vi "ReadINI.vi"(8 "error in (no error)":errorcluster) -> (0 "error out":errorcluster, 3 "value":T1={"TrackQueues?"=TRUE, "ClientTimeout (s)"=30, "LogPath"=path "", "ErrorsToIgnore"=[], "OracleData"={"DBname"="", "User"="", "Password"=""}})   [LabVIEW 2017, in "Server.lvlib"]
uses:
  Server.lvlib
  TypeDefs/ServerINI.ctl
  SubLibs/Oracle/OracleData.ctl
  <vilib>/Utility/error.llb/Error Cluster From Error Code.vi
  <vilib>/ErrorRing/Error Ring.xnode
  SubLibs/Oracle/Oracle.lvlib
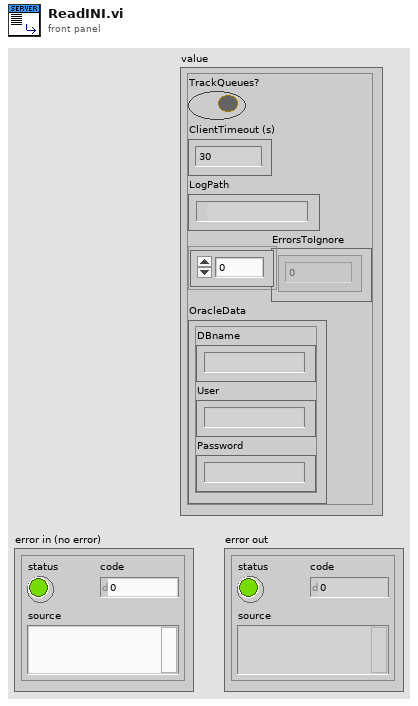
[diagram p1: front panel]
types:
  T1 = typedef "Server.lvlib/ServerINI.ctl" = cluster{"TrackQueues?":bool, "ClientTimeout (s)":u32, "LogPath":path, "ErrorsToIgnore":i32[], "OracleData":T2}
  T2 = typedef "Server.lvlib/Oracle.lvlib/OracleData.ctl" = cluster{"DBname":string, "User":string, "Password":string}
  T3 = enum16{"open", "replace", "create", "open or create", "replace or create", "replace or create with confirmation"}
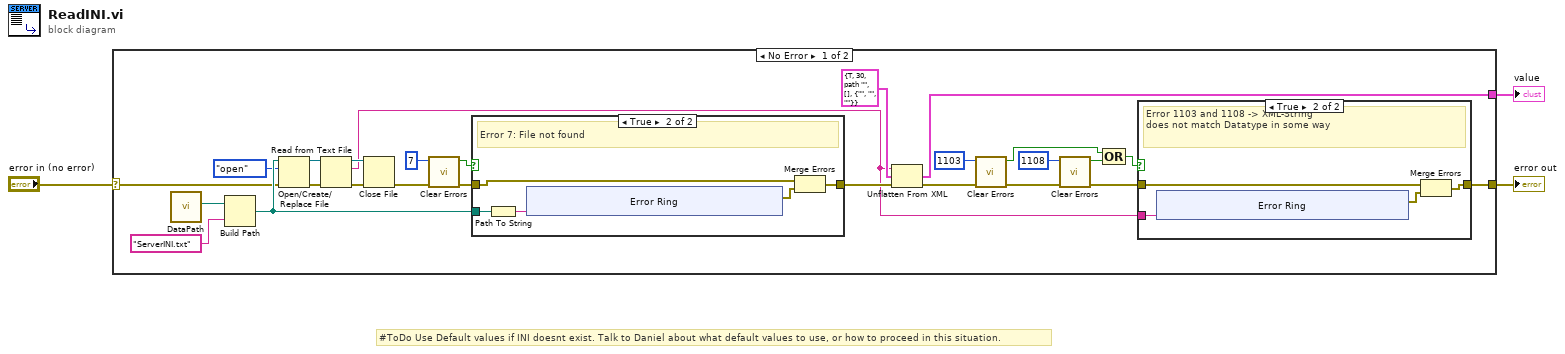
[diagram p0: block diagram]
diagram:
  # "#ToDo Use Default values if INI doesnt exist. Talk to Daniel about what default values to use, or how to proceed in this situation."
  n1 = case shown="No Error" "error in (no error)" {
    selector: "error in (no error)" -> [w14 w55]
    tunnel: [w9 w55] -> w3
    tunnel: [w23 _] -> w2
    frame No Error {
      n2 = call "DataPath.vi"() -> ("DataDirectory"=w21:path)  [unwired: 11 in]
      n3 = Build Path(base path=w21, name or relative path="ServerINI.txt") -> (appended path=w28:path)
      n4 = Open/Create/Replace File(file path (use dialog)=w28, error in=w14, operation (0:open)=T3."open") -> (refnum out=w19:refnum<file>, error out=w16:errorcluster)  [unwired: 3 in, 1 out]
      n5 = Read from Text File(file (use dialog)=w19, error in=w16) -> (refnum out=w20:refnum<file>, text=w8:string, error out=w17:errorcluster)  [unwired: 2 in, 1 out]
      n6 = Close File(refnum=w20, error in=w17) -> (error out=w18:errorcluster)  [unwired: 1 out]
      n7 = call <vilib>:"Clear Errors.vi"("error in (no error)"=w18, "specific error code to clear (0: all)"=7) -> ("error out"=w27:errorcluster, "specific error cleared?"=w26:bool)  [unwired: 4 in]
      n8 = case shown="True" w26 {
        tunnel: w27 -> [w42 w43]
        tunnel: w28 -> [_ w47]
        tunnel: [w42 w44] -> w29
        frame False {
        }
        frame True {
          # "Error 7: File not found"
          n9 = Path To String(path=w47) -> (string=w45:string)
          n10 = xnode "Error Ring"("parameter 0"=w45) -> ("error out"=w46:errorcluster)
          n11 = Merge Errors(w43, w46) -> (w44:errorcluster)
        }
      }
      n12 = Unflatten From XML(xml string=w8, type=T1 {"TrackQueues?"=TRUE, "ClientTimeout (s)"=30, "LogPath"=path "", "ErrorsToIgnore"=[], "OracleData"={"DBname"="", "User"="", "Password"=""}} ("ServerINI"), error in (no error)=w29) -> (value=w23:T1, error out=w11:errorcluster)
      n13 = call <vilib>:"Clear Errors.vi"("error in (no error)"=w11, "specific error code to clear (0: all)"=1103) -> ("error out"=w10:errorcluster, "specific error cleared?"=w13:bool)  [unwired: 4 in]
      n14 = call <vilib>:"Clear Errors.vi"("error in (no error)"=w10, "specific error code to clear (0: all)"=1108) -> ("error out"=w7:errorcluster, "specific error cleared?"=w4:bool)  [unwired: 4 in]
      n15 = Compound Arithmetic op=OR(w13, w4) -> (w5:bool)
      n16 = case shown="True" w5 {
        tunnel: w7 -> [w30 w31]
        tunnel: [w30 w32] -> w9
        tunnel: w8 -> [_ w33]
        frame False {
        }
        frame True {
          # "Error 1103 and 1108 -> XML-String\ndoes not match Datatype in some way"
          n17 = xnode "Error Ring"("parameter 0"=w33) -> ("error out"=w34:errorcluster)
          n18 = Merge Errors(w31, w34) -> (w32:errorcluster)
        }
      }
    }
    frame Error {
    }
  }
  "value" <- w2
  "error out" <- w3
